vi "Stop Core.vi"(10 "final error code":i32, 11 "Sensor in":refnum<class "Sensor.lvclass">) -> (3 "Sensor out":refnum<class "Sensor.lvclass">)   [LabVIEW 2020, in "Sensor.lvlib" / "Sensor.lvclass"]
doc: "(<B>Filename</B>: Actor Framework.lvlib:Actor.lvclass:Stop Core.vi)\n\nDefines what the actor does before it stops. Use the <B>final error code</B> input to determine whether the actor shut down in response to an error.\n\nBy default, this method passes the Stop message along to all auto-stop nested actors. A descendant class may override this method to define additional behavior, such as shutting down any processes the actor initiated in its override of the Actor Core method."
uses:
  Sensor.lvclass
  Sensor.lvclass/Sensor.ctl
  <vilib>/ActorFramework/Actor/Actor.lvclass
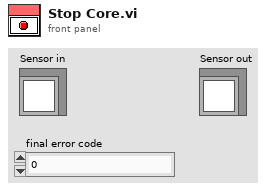
[diagram p1: front panel]
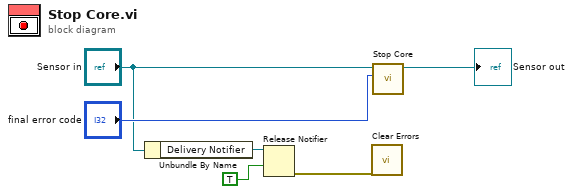
[diagram p0: block diagram]
diagram:
  n1 = Unbundle By Name("Sensor in") -> ("Delivery Notifier"=w3:refnum<notifier>)
  n2 = Release Notifier(notifier=w3, force destroy? (F)=TRUE) -> (error out=w1:errorcluster)  [unwired: 1 in, 2 out]
  n3 = call <vilib>:"Clear Errors.vi"("error in (no error)"=w1) -> ()  [unwired: 5 in, 2 out]
  n4 = call-parent "Stop Core.vi"("final error code"="final error code", "Actor in"="Sensor in") -> ("Actor out"=→"Sensor out":refnum<class "Sensor.lvclass">)  [unwired: 9 in]
